vi "mainActivity__viAdd.vi"(8 "error in":errorcluster, 11 "VI":path) -> (0 "error out":errorcluster)   [LabVIEW 2014]
uses:
  glb/glb_static.vi
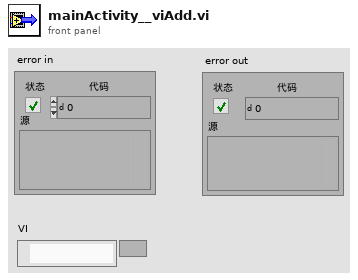
[diagram p1: front panel]
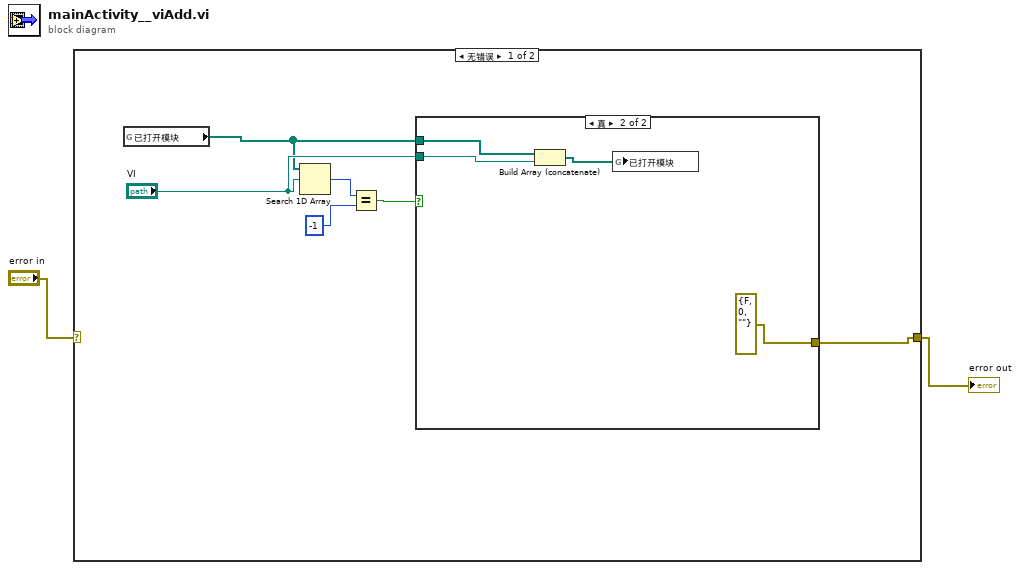
[diagram p0: block diagram]
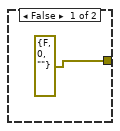
[diagram p2: hidden frame]
diagram:
  n1 = case shown="无错误" "error in" {
    selector: "error in" -> [_ w14]
    tunnel: [w5 w14] -> w1
    frame No Error {
      n2 = global read "glb_static.vi" "已打开模块"() -> (w3:path[])
      n3 = Search 1D Array(1D array=w3, element="VI") -> (index of element=w8:i32)  [unwired: 1 in]
      n4 = Equal?(x=w8, y=-1 ("元素索引")) -> (x = y?=w6:bool)
      n5 = case shown="真" w6 {
        tunnel: w3 -> [_ w11]
        tunnel: "VI" -> [_ w12]
        tunnel: [errorcluster {"status"=FALSE, "code"=0, "source"=""} ("错误常量") errorcluster {"status"=FALSE, "code"=0, "source"=""} ("错误常量")] -> w5
        frame False {
        }
        frame True {
          n6 = Build Array (concatenate)(w11, w12) -> (w10:path[])
          n7 = global write "glb_static.vi" "已打开模块"(w10) -> ()
        }
      }
    }
    frame Error {
    }
  }
  "error out" <- w1
